vi "offline analyzerV2.vi"() -> ()   [LabVIEW 2017]
uses:
  <vilib>/Utility/file.llb/Read Delimited Spreadsheet (I64).vi
  <vilib>/Utility/file.llb/Write Delimited Spreadsheet (string).vi
  <vilib>/Utility/file.llb/Write Delimited Spreadsheet (DBL).vi
panel:
  out "appended path":path=path "G:/tdc/2017/test_20240423_023818_single_csv.csv"
  in  "col":i32
  in  "file path (dialog if empty)":path=path "G:/tdc/2017/code_density_rom.mem"
  out "size(s)":i32[](array[numeric])=[2048, 128]
  out "Array":u32[][](array[numeric]) format="%x"
  out "cal":u32[][](graph)
  out "x/y":dbl=0.025
  out "index":i32=393690
  out "time":dbl=49958037665847.64 format="%.000f"
  in  "通道数量":i32=128
  out "fine":u64=801 format="%x"
  out "data 5":string
  in  "codeDensity":path=path "G:/tdc/2017/test_20240423_093608_codeDensity.csv"
  out "file path (dialog if empty) 2":path=path "G:/tdc/2017/test_20240423_023818_multiple_csv.csv"
  out "ip":u64=35 format="%x"
  out "data 9":string="#"
  out "result string":string="test_20240423_023818"
  out "sent number":u64=49211 format="%x"
  out "trigger number":u64=49958 format="%x"
  out "data 8":string="Ã&"
  out "data 7":string="À;"
  out "data":dbl[](array[numeric])=[0.0, 0.0, 0.0, 0.0, 0.0, 49958037665847.64, 0.0, 0.0, 0.0, 0.0, 0.0, 0.0, 0.0, 0.0, 0.0, 0.0, 0.0, 0.0, 0.0, 0.0, 0.0, 0.0, 0.0, 0.0, 0.0, 0.0, 0.0, 0.0, 0.0, 0.0, 0.0, 0.0, 0.0, 0.0, 0.0, 0.0, 0.0, 0.0, 0.0, 0.0, 0.0, 0.0, 0.0, 0.0, 0.0, 0.0, 0.0, 0.0, 0.0, 0.0, 0.0, 0.0, 0.0, 0.0, 0.0, 0.0, 0.0, 0.0, 0.0, 0.0, 0.0, 0.0, 0.0, 0.0, 0.0, 0.0, 0.0, 0.0, 0.0, 0.0, 0.0, 0.0, 0.0, 0.0, 0.0, 0.0, 0.0, 0.0, 0.0, 0.0, 0.0, 0.0, 0.0, 0.0, 0.0, 0.0, 0.0, 0.0, 0.0, 0.0, 0.0, 0.0, 0.0, 0.0, 0.0, 0.0, 0.0, 0.0, 0.0, 0.0, 0.0, 0.0, 0.0, 0.0, 0.0, 0.0, 0.0, 0.0, 0.0, 0.0, 0.0, 0.0, 0.0, 0.0, 0.0, 0.0, 0.0, 0.0, 0.0, 0.0, 0.0, 0.0, 0.0, 0.0, 0.0, 0.0, 0.0, 0.0]
  out "data 2":string
  out "data 4":string
  out "coarse time":u64=19983215066 format="%x"
  out "error out":errorcluster
  out "substring":string="…"
  out "number 3":u32
  out "channel number":u64=5 format="%x"
  in  "channel":u64
  out "data 6":string
  out "data 3":string="Z"
  in  "dat file (use dialog)":path=path "G:/tdc/2017/test_20240423_023818.dat"
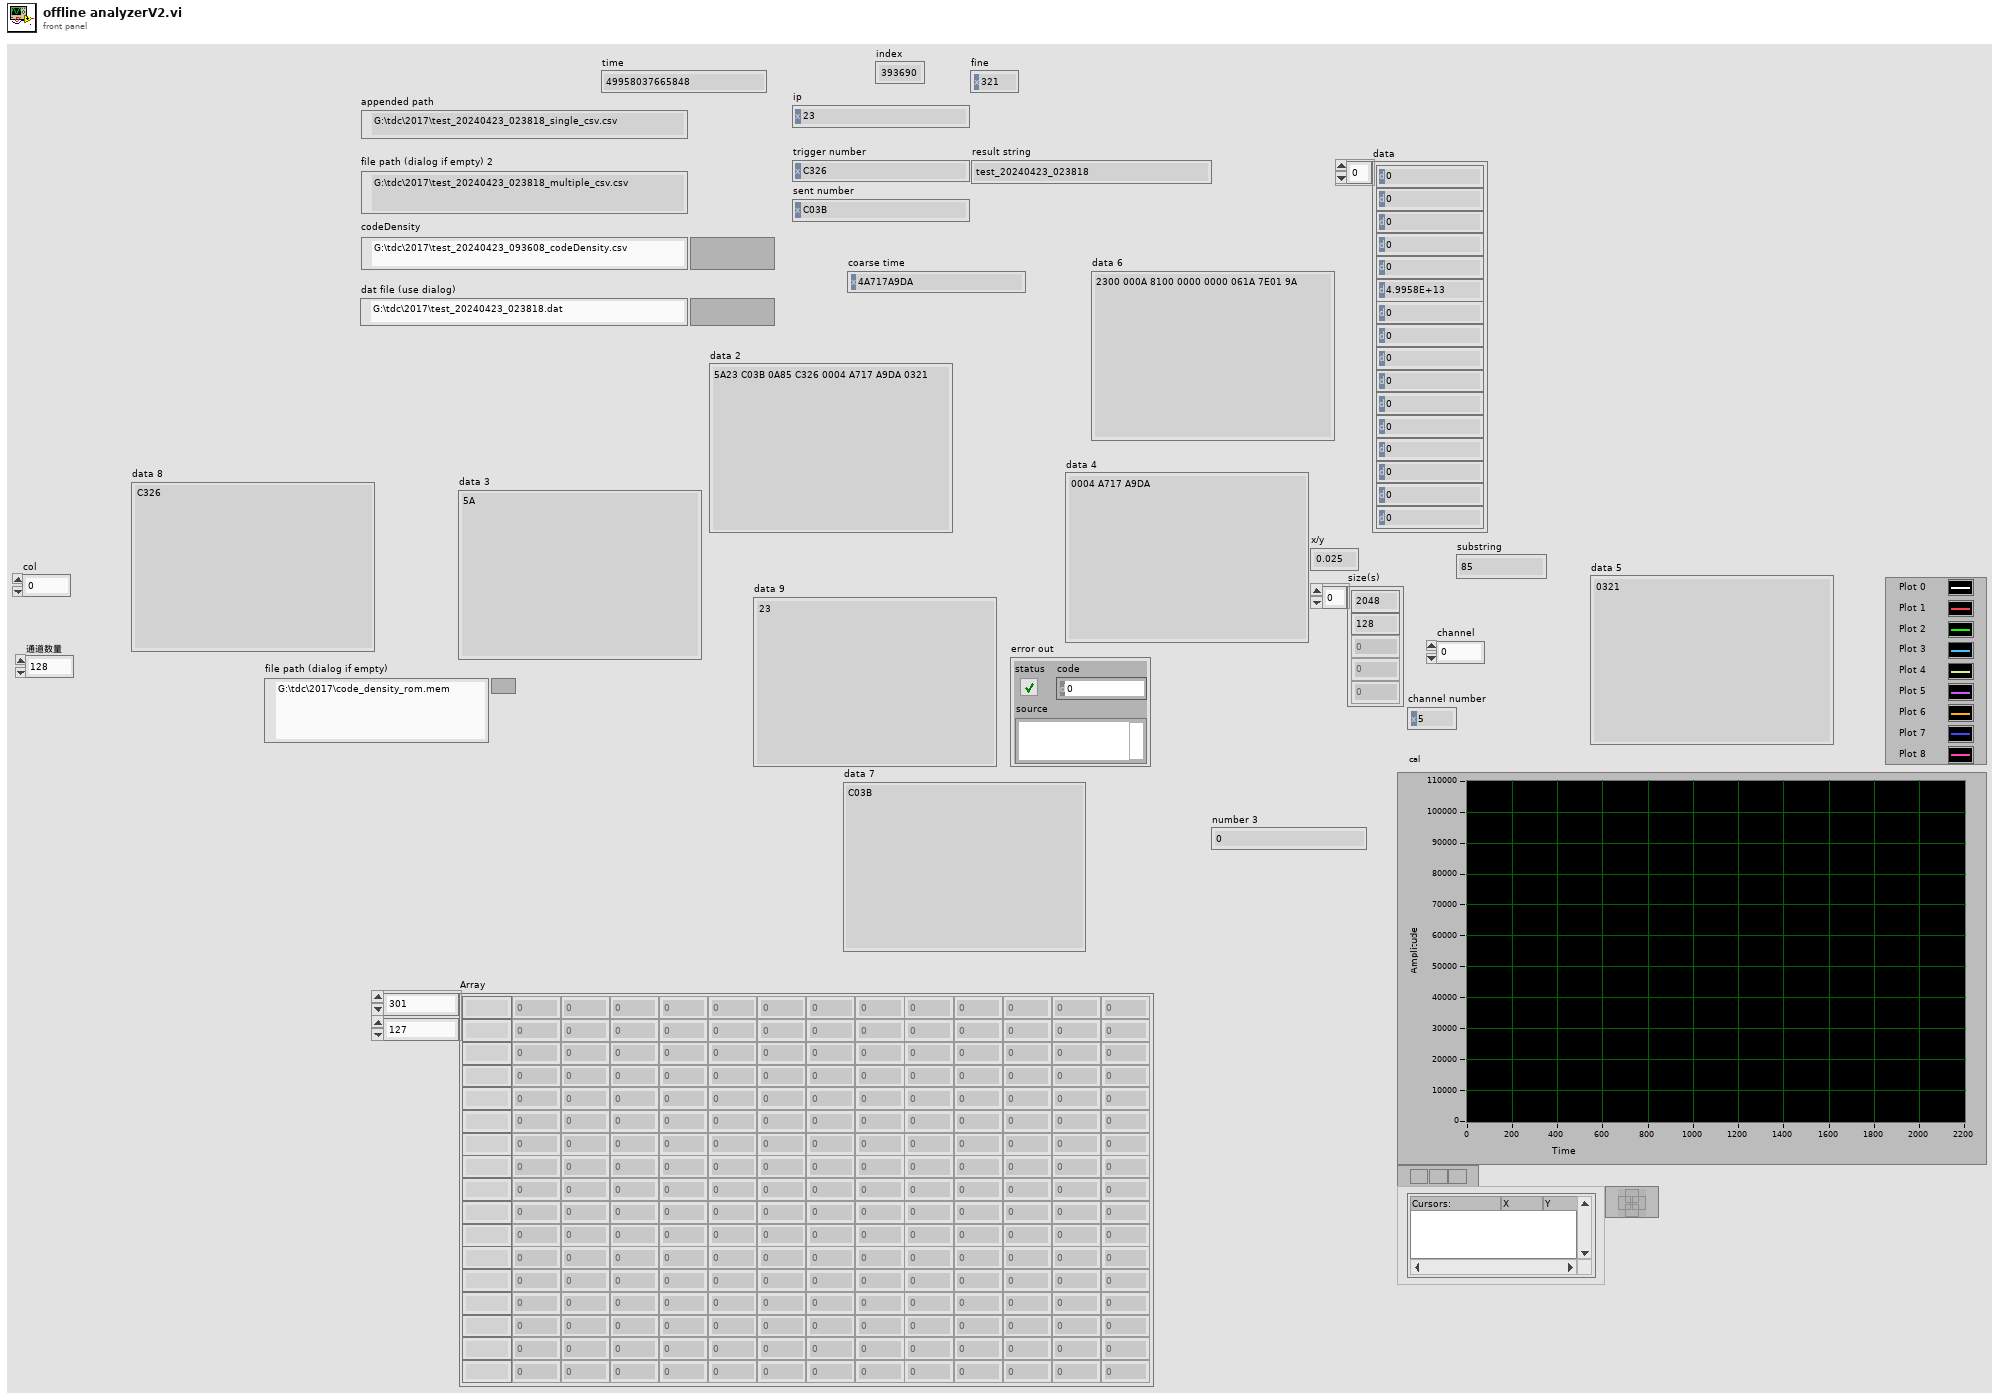
[diagram p1: front panel]
types:
  T1 = enum16{"open", "replace", "create", "open or create", "replace or create", "replace or create with confirmation"}
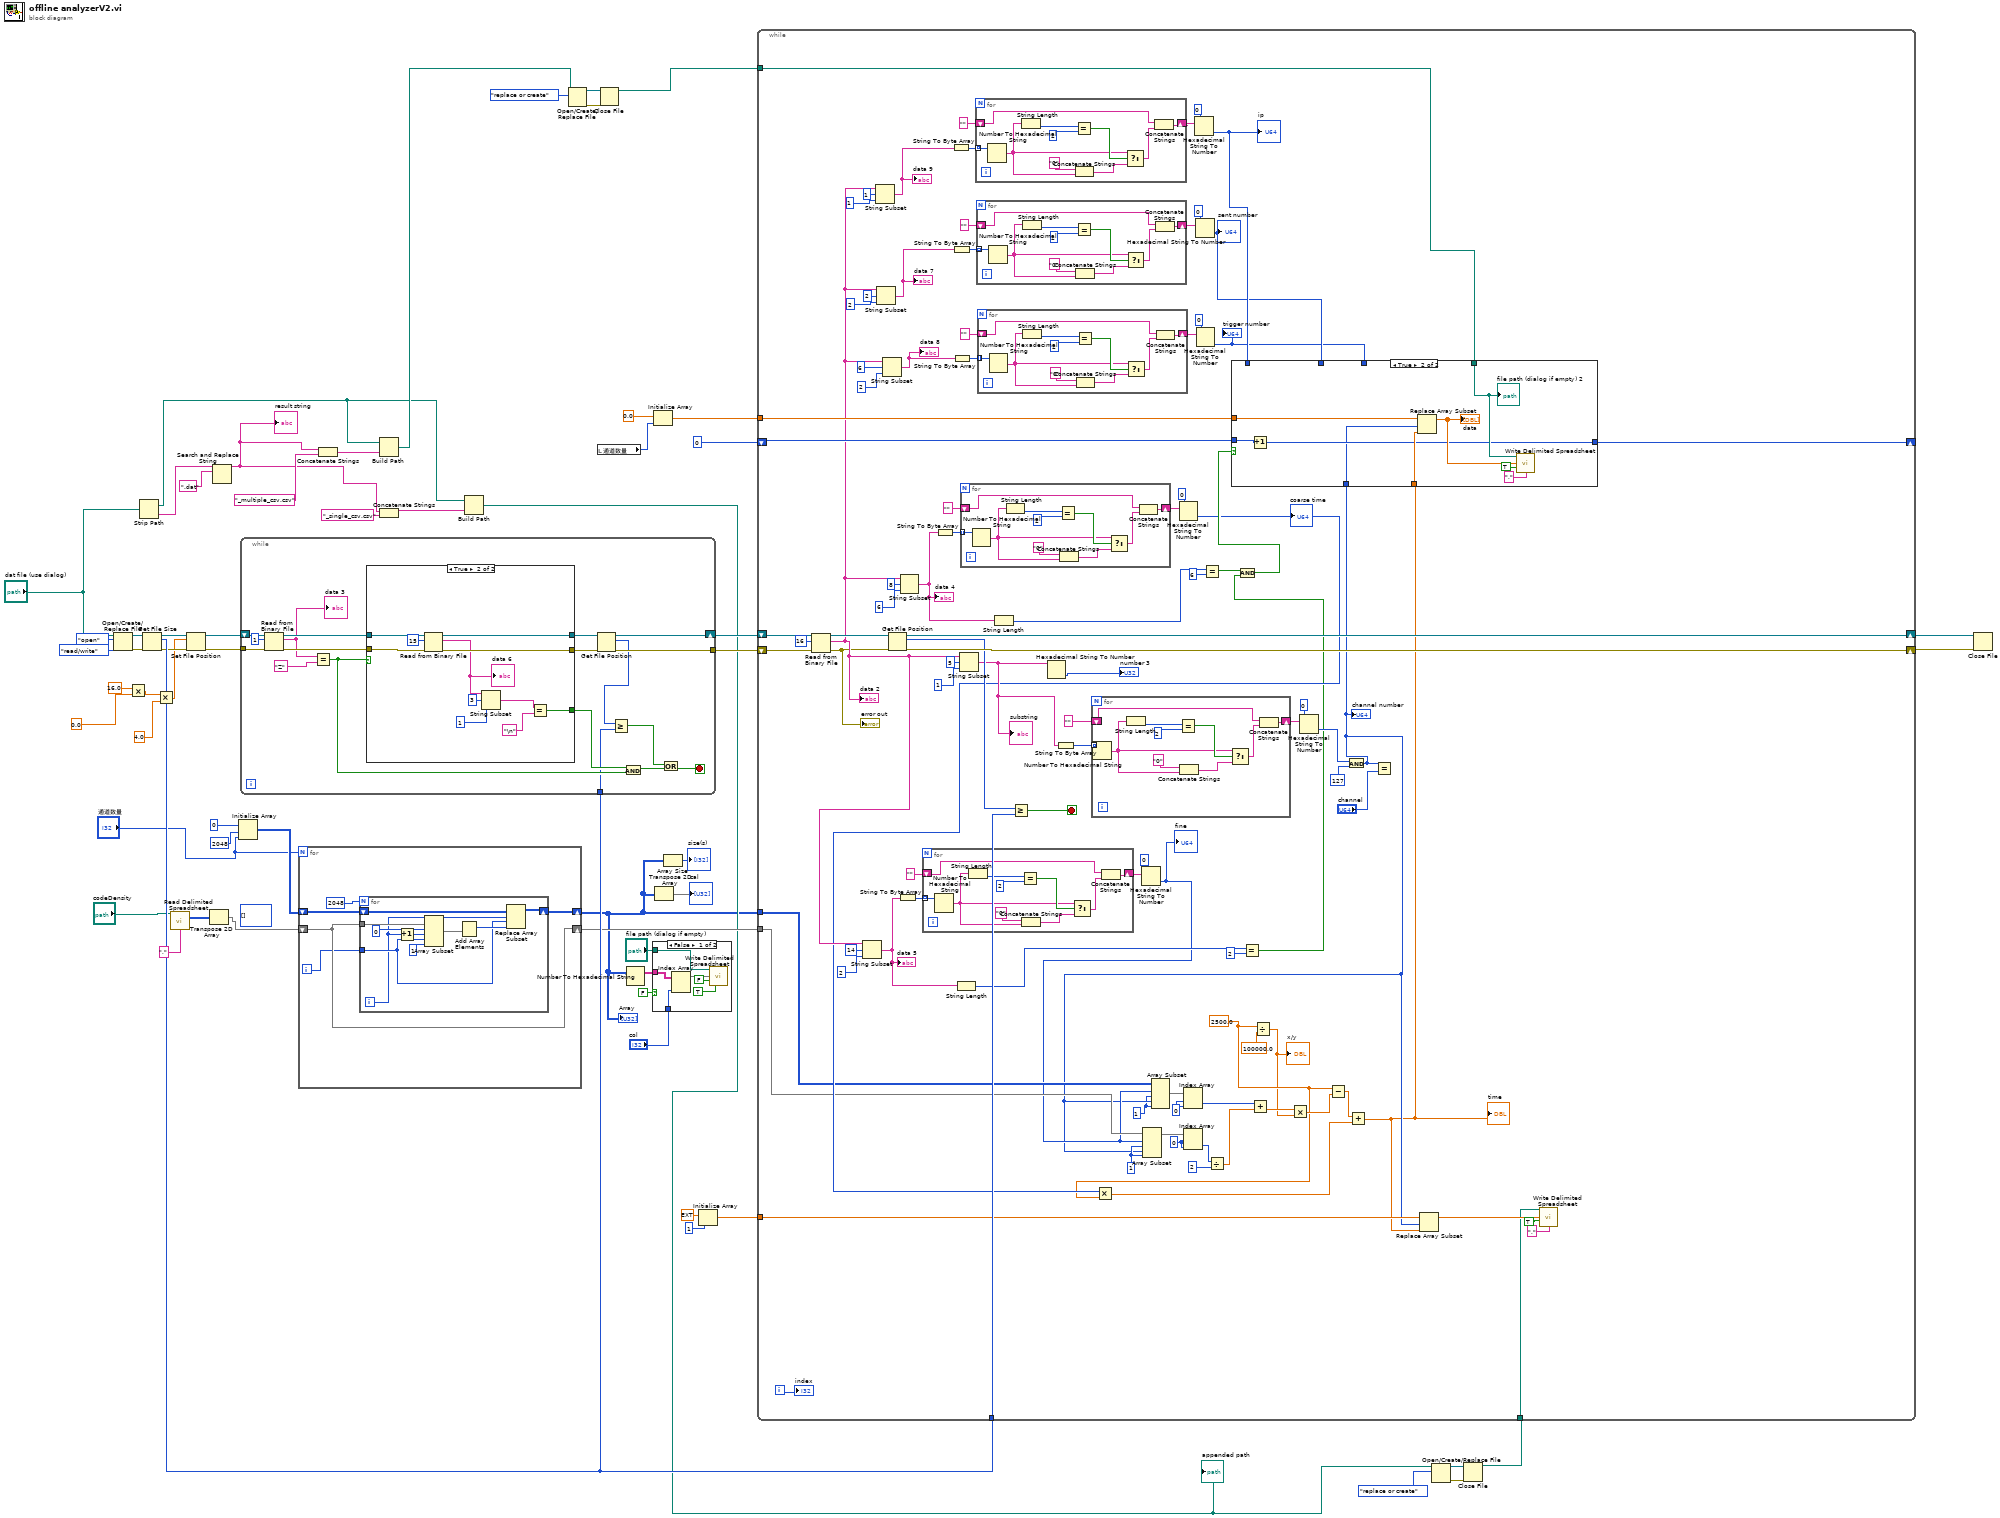
[diagram p0: block diagram]
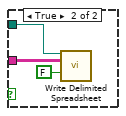
[diagram p2: hidden frame]
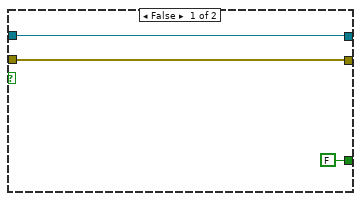
[diagram p4: hidden frame]
diagram:
  (unwired) i64[][] []
  n1 = Open/Create/Replace File(file path (use dialog)="dat file (use dialog)", operation (0:open)=T1."open", access (0:read/write)=enum16{"read/write", "read-only", "write-only"}."read/write") -> (refnum out=w60:refnum<file>, error out=w55:errorcluster)  [unwired: 3 in, 1 out]
  n2 = Multiply(x=16.0, y=0.0) -> (x*y=w25:dbl)
  n3 = Strip Path(path="dat file (use dialog)") -> (stripped path=w14:path, name=w49:string)
  n4 = Get File Size(file=w60, error in=w55) -> (refnum out=w31:refnum<file>, size (in bytes)=w51:i64, 0:w29:errorcluster)
  n5 = Multiply(x=w25, y=4.0) -> (x*y=w23:dbl)
  n6 = call-poly <vilib>:"Read Delimited Spreadsheet.vi"("file path (dialog if empty)"="codeDensity", "delimiter (\\t)"="," ("delimiter (\\t)")) -> ("all rows"=w1:i64[][])  [unwired: 8 in, 5 out]
  n7 = Set File Position(offset (in bytes) (0)=w23, refnum=w31, error in=w29) -> (refnum out=w30:refnum<file>, error out=w28:errorcluster)  [unwired: 1 in]
  n8 = Transpose 2D Array(2D array=w1) -> (transposed array=w36:i64[][])
  n9 = Search and Replace String(input string=w49, search string=".dat") -> (result string=w16:string)  [unwired: 6 in, 3 out]
  "result string" <- w16
  n10 = Initialize Array(u32 0 ("element"), 2048 ("dimension size"), "通道数量") -> (w37:u32[][])
  n11 = while {
    tunnel: w28 -> [w77]
    shift-right: [w65] -> w56
    shift-left: w30 -> [w78]
    tunnel: [w66] -> w57
    tunnel: w51 -> [w64]
    stop <- w62 stop-if-true
    n12 = Read from Binary File(8:w77, 10:1 ("count (1)"), 11:w78) -> (0:w73:errorcluster, 2:w71:string, 3:w74:refnum<file>)  [unwired: 3 in, 1 out]
    "data 3" <- w71
    n13 = Equal?(x=w71, y="Z") -> (x = y?=w68:bool)
    n14 = case shown="True" w68 {
      tunnel: w74 -> [w81 w92]
      tunnel: w73 -> [w80 w91]
      tunnel: [w81 w89] -> w72
      tunnel: [w80 w88] -> w67
      tunnel: [FALSE w82] -> w69
      frame False {
      }
      frame True {
        n15 = Read from Binary File(8:w91, 10:15 ("count (1)"), 11:w92) -> (0:w88:errorcluster, 2:w85:string, 3:w89:refnum<file>)  [unwired: 3 in, 1 out]
        "data 6" <- w85
        n16 = String Subset(string=w85, offset (0)=3, length (rest)=1 ("length (rest)")) -> (substring=w84:string)
        n17 = Equal?(x=w84, y="\n") -> (x = y?=w82:bool)
      }
    }
    n18 = Get File Position(4:w67, 7:w72) -> (0:w66:errorcluster, 2:w63:i64, 3:w65:refnum<file>)
    n19 = Greater Or Equal?(x=w63, y=w64) -> (x >= y?=w61:bool)
    n20 = Compound Arithmetic op=AND(w69, w68) -> (w70:bool)
    n21 = Or(x=w61, y=w70) -> (x .or. y?=w62:bool)
  }
  n22 = for {
    N: "通道数量" -> [_]
    shift-right: [w95] -> w9
    shift-left: w37 -> [w96]
    shift-right: [w94] -> w43
    shift-left: w36 -> [w94]
    i -> [w93]
    n23 = for {
      N: 2048 -> [_]
      tunnel: w94 -> [w107]
      tunnel: w93 -> [w100]
      shift-right: [w102] -> w95
      shift-left: w96 -> [w103]
      i -> [w99]
      n24 = Increment(x=w99) -> (x+1=w98:i32)
      n25 = Array Subset(array=w107, index (row)=0 ("索引"), length (row)=w98, index (col)=w100, length (col)=1 ("长度")) -> (w104:i64[][])
      n26 = Add Array Elements(numeric array=w104) -> (sum=w101:i64)
      n27 = Replace Array Subset(array=w103, new element=w101, index (row)=w99, index (col)=w100) -> (w102:u32[][])
    }
  }
  "Array" <- w9
  n28 = Concatenate Strings(w16, "_multiple_csv.csv" ("string")) -> (w46:string)
  n29 = Build Path(base path=w14, name or relative path=w46) -> (appended path=w19:path)
  n30 = Concatenate Strings(w16, "_single_csv.csv" ("string")) -> (w15:string)
  n31 = Build Path(base path=w14, name or relative path=w15) -> (appended path=w13:path)
  "appended path" <- w13
  n32 = Open/Create/Replace File(file path (use dialog)=w19, operation (0:open)=T1."replace or create") -> (refnum out=w20:refnum<file>, error out=w21:errorcluster)  [unwired: 4 in, 1 out]
  n33 = local read "通道数量"() -> (w2:i32)
  n34 = Close File(refnum=w20, error in=w21) -> (path=w18:path)  [unwired: 1 out]
  n35 = Number To Hexadecimal String(2:w9) -> (0:w8:string[][])  [unwired: 1 in]
  n36 = case shown="False" FALSE {
    tunnel: "file path (dialog if empty)" -> [w112 w116]
    tunnel: w8 -> [w111 w114]
    tunnel: "col" -> [w109 _]
    frame False {
      n37 = Index Array(array=w111, index (col)=w109) -> (element=w110:string[])  [unwired: 1 in]
      n38 = call-poly <vilib>:"Write Delimited Spreadsheet.vi"("file path (dialog if empty)"=w112, "1D data"=w110, "append to file? (new file:F)"=FALSE, "transpose? (no:F)"=TRUE) -> ()  [unwired: 10 in, 2 out]
    }
    frame True {
      n39 = call-poly <vilib>:"Write Delimited Spreadsheet.vi"("file path (dialog if empty)"=w116, "2D data"=w114, "append to file? (new file:F)"=FALSE) -> ()  [unwired: 11 in, 2 out]
    }
  }
  n40 = Initialize Array(0.0 ("element"), w2) -> (w3:dbl[])
  n41 = Transpose 2D Array(2D array=w9) -> (transposed array=→"cal":u32[][])
  n42 = Array Size(array=w9) -> (size(s)=→"size(s)":i32[])
  n43 = Initialize Array(ext 0.0 ("element"), 1 ("dimension size")) -> (w40:ext[])
  n44 = Open/Create/Replace File(file path (use dialog)=w13, operation (0:open)=T1."replace or create") -> (refnum out=w33:refnum<file>, error out=w34:errorcluster)  [unwired: 4 in, 1 out]
  n45 = Close File(refnum=w33, error in=w34) -> (path=w32:path)  [unwired: 1 out]
  n46 = while {
    shift-right: [w211] -> w54
    shift-left: w56 -> [w215]
    shift-right: [w213] -> w53
    shift-left: w57 -> [w216]
    tunnel: w51 -> [w209]
    shift-right: [w158] -> _
    shift-left: 0 ("length (rest)") -> [w189]
    tunnel: w18 -> [w159]
    tunnel: w9 -> [w132]
    tunnel: w43 -> [w133]
    tunnel: w40 -> [w128]
    tunnel: w32 -> [w120]
    tunnel: w3 -> [w188]
    i -> [w119]
    stop <- w208 stop-if-true
    w121 = 0 ("index (row)")
    w123 = 1 ("长度")
    w135 = 2500.0 ("x")
    w149 = 0 ("索引 (行)")
    w151 = 1 ("长度")
    n47 = Read from Binary File(8:w216, 10:16 ("count (1)"), 11:w215) -> (0:w117:errorcluster, 2:w137:string, 3:w212:refnum<file>)  [unwired: 3 in, 1 out]
    "data 2" <- w137
    "error out" <- w117
    n48 = String Subset(string=w137, offset (0)=14, length (rest)=2 ("length (rest)")) -> (substring=w140:string)
    "data 5" <- w140
    n49 = String Subset(string=w137, offset (0)=1, length (rest)=1 ("length (rest)")) -> (substring=w169:string)
    "data 9" <- w169
    n50 = String Subset(string=w137, offset (0)=2, length (rest)=2 ("length (rest)")) -> (substring=w170:string)
    "data 7" <- w170
    n51 = String Subset(string=w137, offset (0)=6, length (rest)=2 ("length (rest)")) -> (substring=w175:string)
    "data 8" <- w175
    n52 = Get File Position(4:w117, 7:w212) -> (0:w213:errorcluster, 2:w210:i64, 3:w211:refnum<file>)
    n53 = String To Byte Array(string=w140) -> (unsigned byte array=w143:u8[])
    n54 = String Subset(string=w137, offset (0)=8, length (rest)=6 ("length (rest)")) -> (substring=w186:string)
    "data 4" <- w186
    n55 = for {
      shift-right: [w225] -> w142
      shift-left: "" ("format string") -> [w222]
      tunnel: w143 -> [w226] mode=indexing
      n56 = Number To Hexadecimal String(2:w226) -> (0:w218:string)  [unwired: 1 in]
      n57 = String Length(string=w218) -> (length=w224:i32)
      n58 = Equal?(x=w224, y=2) -> (x = y?=w221:bool)
      n59 = Concatenate Strings("0" ("format string"), w218) -> (w220:string)
      n60 = Select(t=w218, s=w221, f=w220) -> (s? t:f=w217:string)
      n61 = Concatenate Strings(w222, w217) -> (w225:string)
    }
    n62 = String To Byte Array(string=w186) -> (unsigned byte array=w204:u8[])
    n63 = String To Byte Array(string=w169) -> (unsigned byte array=w166:u8[])
    n64 = String To Byte Array(string=w170) -> (unsigned byte array=w173:u8[])
    n65 = String To Byte Array(string=w175) -> (unsigned byte array=w177:u8[])
    n66 = String Length(string=w140) -> (length=w139:i32)
    n67 = String Subset(string=w137, offset (0)=5, length (rest)=1 ("length (rest)")) -> (substring=w192:string)
    "substring" <- w192
    n68 = for {
      shift-right: [w285] -> w203
      shift-left: "" ("format string") -> [w282]
      tunnel: w204 -> [w286] mode=indexing
      n69 = Number To Hexadecimal String(2:w286) -> (0:w278:string)  [unwired: 1 in]
      n70 = String Length(string=w278) -> (length=w284:i32)
      n71 = Equal?(x=w284, y=2) -> (x = y?=w281:bool)
      n72 = Concatenate Strings("0" ("format string"), w278) -> (w280:string)
      n73 = Select(t=w278, s=w281, f=w280) -> (s? t:f=w277:string)
      n74 = Concatenate Strings(w282, w277) -> (w285:string)
    }
    n75 = for {
      shift-right: [w235] -> w167
      shift-left: "" ("format string") -> [w232]
      tunnel: w166 -> [w236] mode=indexing
      n76 = Number To Hexadecimal String(2:w236) -> (0:w228:string)  [unwired: 1 in]
      n77 = String Length(string=w228) -> (length=w234:i32)
      n78 = Equal?(x=w234, y=2) -> (x = y?=w231:bool)
      n79 = Concatenate Strings("0" ("format string"), w228) -> (w230:string)
      n80 = Select(t=w228, s=w231, f=w230) -> (s? t:f=w227:string)
      n81 = Concatenate Strings(w232, w227) -> (w235:string)
    }
    n82 = for {
      shift-right: [w245] -> w172
      shift-left: "" ("format string") -> [w242]
      tunnel: w173 -> [w246] mode=indexing
      n83 = Number To Hexadecimal String(2:w246) -> (0:w238:string)  [unwired: 1 in]
      n84 = String Length(string=w238) -> (length=w244:i32)
      n85 = Equal?(x=w244, y=2) -> (x = y?=w241:bool)
      n86 = Concatenate Strings("0" ("format string"), w238) -> (w240:string)
      n87 = Select(t=w238, s=w241, f=w240) -> (s? t:f=w237:string)
      n88 = Concatenate Strings(w242, w237) -> (w245:string)
    }
    n89 = for {
      shift-right: [w255] -> w178
      shift-left: "" ("format string") -> [w252]
      tunnel: w177 -> [w256] mode=indexing
      n90 = Number To Hexadecimal String(2:w256) -> (0:w248:string)  [unwired: 1 in]
      n91 = String Length(string=w248) -> (length=w254:i32)
      n92 = Equal?(x=w254, y=2) -> (x = y?=w251:bool)
      n93 = Concatenate Strings("0" ("format string"), w248) -> (w250:string)
      n94 = Select(t=w248, s=w251, f=w250) -> (s? t:f=w247:string)
      n95 = Concatenate Strings(w252, w247) -> (w255:string)
    }
    n96 = String Length(string=w186) -> (length=w184:i32)
    n97 = Greater Or Equal?(x=w210, y=w209) -> (x >= y?=w208:bool)
    n98 = Hexadecimal String To Number(string=w192) -> (number=→"number 3":u32)  [unwired: 2 in, 1 out]
    n99 = String To Byte Array(string=w192) -> (unsigned byte array=w195:u8[])
    n100 = for {
      shift-right: [w275] -> w194
      shift-left: "" ("format string") -> [w272]
      tunnel: w195 -> [w276] mode=indexing
      n101 = Number To Hexadecimal String(2:w276) -> (0:w268:string)  [unwired: 1 in]
      n102 = String Length(string=w268) -> (length=w274:i32)
      n103 = Equal?(x=w274, y=2) -> (x = y?=w271:bool)
      n104 = Concatenate Strings("0" ("format string"), w268) -> (w270:string)
      n105 = Select(t=w268, s=w271, f=w270) -> (s? t:f=w267:string)
      n106 = Concatenate Strings(w272, w267) -> (w275:string)
    }
    n107 = Hexadecimal String To Number(string=w142, default (0uL)=u64 0 ("default (0 U32)")) -> (number=w130:u64)  [unwired: 1 in, 1 out]
    "fine" <- w130
    n108 = Hexadecimal String To Number(string=w203, default (0uL)=u64 0 ("default (0 U32)")) -> (number=w136:u64)  [unwired: 1 in, 1 out]
    "coarse time" <- w136
    n109 = Multiply(x=w136, y=w135) -> (x*y=w153:dbl)
    n110 = Hexadecimal String To Number(string=w167, default (0uL)=u64 0 ("default (0 U32)")) -> (number=w162:u64)  [unwired: 1 in, 1 out]
    "ip" <- w162
    n111 = Hexadecimal String To Number(string=w172, default (0uL)=u64 0 ("default (0 U32)")) -> (number=w161:u64)  [unwired: 1 in, 1 out]
    "sent number" <- w161
    n112 = Hexadecimal String To Number(string=w178, default (0uL)=u64 0 ("default (0 U32)")) -> (number=w160:u64)  [unwired: 1 in, 1 out]
    "trigger number" <- w160
    n113 = Equal?(x=w184, y=6) -> (x = y?=w185:bool)
    n114 = Equal?(x=w139, y=2) -> (x = y?=w131:bool)
    n115 = And(x=w185, y=w131) -> (x .and. y?=w182:bool)
    n116 = Divide(x=w135, y=100000.0) -> (x/y=w134:dbl)
    "x/y" <- w134
    n117 = Hexadecimal String To Number(string=w194, default (0uL)=u64 0 ("default (0 U32)")) -> (number=w191:u64)  [unwired: 1 in, 1 out]
    n118 = And(x=w191, y=u64 127 ("default (0 U32)")) -> (x .and. y?=w127:u64)
    "channel number" <- w127
    n119 = Array Subset(array=w133, index (row)=w130, length (row)=w151, index (col)=w127, length (col)=w151) -> (w150:i64[][])
    n120 = Array Subset(array=w132, index (row)=w130, length (row)=w123, index (col)=w127, length (col)=w123) -> (w122:u32[][])
    n121 = Index Array(array=w122, index (row)=w121, index (col)=w121) -> (element=w155:u32)
    n122 = Index Array(array=w150, index (row)=w149, index (col)=w149) -> (element=w148:i64)
    n123 = Divide(x=w148, y=u32 2) -> (x/y=w152:dbl)
    n124 = Add(x=w155, y=w152) -> (x+y=w154:dbl)
    n125 = Multiply(x=w154, y=w134) -> (x*y=w147:dbl)
    n126 = Subtract(x=w135, y=w147) -> (x-y=w118:dbl)
    n127 = Add(x=w118, y=w153) -> (x+y=w126:dbl)
    "time" <- w126
    n128 = case shown="True" w182 {
      tunnel: w189 -> [w257 w262]
      tunnel: w188 -> [_ w259]
      tunnel: w126 -> [_ w263]
      tunnel: w162 -> [_ _]
      tunnel: w161 -> [_ _]
      tunnel: w160 -> [_ _]
      tunnel: w127 -> [_ w258]
      tunnel: w159 -> [_ w265]
      tunnel: [w257 w261] -> w158
      frame False {
      }
      frame True {
        n129 = Increment(x=w262) -> (x+1=w261:i32)
        n130 = Replace Array Subset(array=w259, new element=w263, index=w258) -> (w264:dbl[])
        "data" <- w264
        n131 = call-poly <vilib>:"Write Delimited Spreadsheet.vi"("file path (dialog if empty)"=w265, "1D data"=w264, "append to file? (new file:F)"=TRUE, "delimiter (\\t)"="," ("delimiter (\\t)")) -> ()  [unwired: 10 in, 2 out]
        "file path (dialog if empty) 2" <- w265
      }
    }
    n132 = Equal?(x=w127, y="channel") -> ()  [unwired: 1 out]
    n133 = Replace Array Subset(array=w128, new element=w126, index=w127) -> (w125:ext[])
    n134 = call-poly <vilib>:"Write Delimited Spreadsheet.vi"("file path (dialog if empty)"=w120, "1D data"=w125, "append to file? (new file:F)"=TRUE, "delimiter (\\t)"="," ("delimiter (\\t)")) -> ()  [unwired: 10 in, 2 out]
    "index" <- w119
  }
  n135 = Close File(refnum=w54, error in=w53) -> ()  [unwired: 2 out]
